vi "Caller.vi"   [LabVIEW 2015]
uses:
  Lib.lvlib
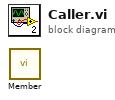
[diagram p0: block diagram]
diagram:
  n1 = call "Member.vi"() -> ()  [unwired: 12 in]
